vi "tmp_toml_file_write.vi"(8 "error in (no error)":errorcluster, 9 "text":string, 10 "operation (replace or create)":T1(ring)=enum."replace or create", 11 "path":path) -> (0 "error out":errorcluster)   [LabVIEW 2017]
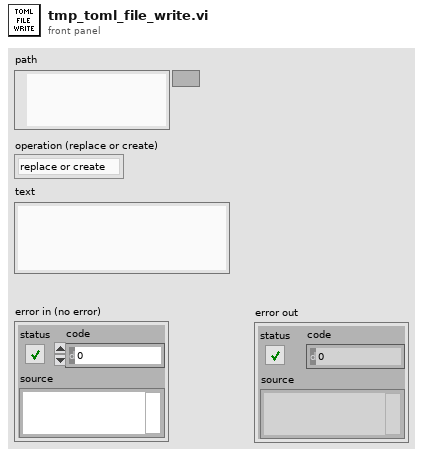
[diagram p1: front panel]
types:
  T1 = enum16{"open", "replace", "create", "open or create", "replace or create", "replace or create with confirmation"}
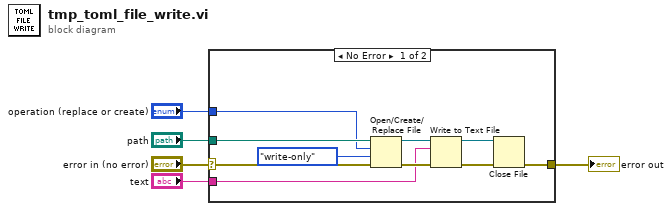
[diagram p0: block diagram]
diagram:
  n1 = case shown="No Error" "error in (no error)" {
    selector: "error in (no error)" -> [w15 w16]
    tunnel: "path" -> [w14 _]
    tunnel: [w13 w16] -> w3
    tunnel: "operation (replace or create)" -> [w12 _]
    tunnel: "text" -> [w6 _]
    frame No Error {
      n2 = Open/Create/Replace File(file path (use dialog)=w14, error in=w15, operation (0:open)=w12, access (0:read/write)=enum16{"read/write", "read-only", "write-only"}."write-only") -> (refnum out=w10:refnum<file>, error out=w9:errorcluster)  [unwired: 2 in, 1 out]
      n3 = Write to Text File(file (use dialog)=w10, text=w6, error in=w9) -> (refnum out=w7:refnum<file>, error out=w8:errorcluster)  [unwired: 1 in, 1 out]
      n4 = Close File(refnum=w7, error in=w8) -> (error out=w13:errorcluster)  [unwired: 1 out]
    }
    frame Error {
    }
  }
  "error out" <- w3
